vi "Demo.vi"   [LabVIEW 2020, in "Icon Decorator.lvclass"]
uses:
  Icon Decorator.lvclass
  Result Types/Assertion Result/Public/TypeDefs/Status.ctl
  Result Types/Assertion Result/Assertion Result.lvlib
types:
  T1 = typedef "Assertion Result.lvlib/Status.ctl" = enum16{"Pass", "Fail", "Error", "Skipped", "Setup Error", "Broken", "Teardown Error"}
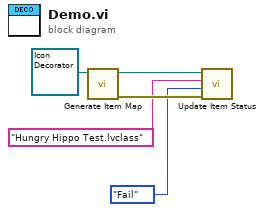
[diagram p0: block diagram]
diagram:
  n1 = call "Generate Item Map.vi"("Icon Decorator In"=refnum<class "Icon Decorator.lvclass"> refnum) -> ("error out"=w4:errorcluster, "Icon Decorator Out"=w5:refnum<class "Icon Decorator.lvclass">)  [unwired: 9 in]
  n2 = call "Update Item Status.vi"("error in (no error)"=w4, "Status"=Status."Fail", "Test Case"="Hungry Hippo Test.lvclass", "Icon Decorator In"=w5) -> ()  [unwired: 6 in, 2 out]
